vi "ReceiveFloat.vi"(6 "Timeout ms":i32=1, 7 "UDP Input":T1) -> (0 "Error Out":errorcluster, 1 "Received Data":dbl, 2 "Did Receive":bool, 3 "UDP Output":T1)   [LabVIEW 2019]
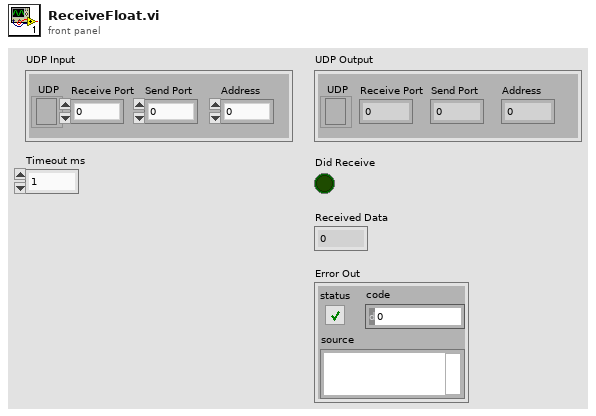
[diagram p1: front panel]
types:
  T1 = cluster{"UDP":refnum<k16>, "Receive Port":i32, "Send Port":i32, "Address":i64}
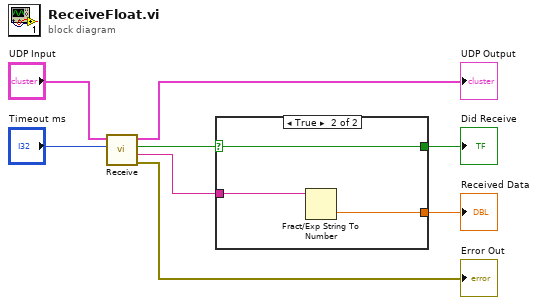
[diagram p0: block diagram]
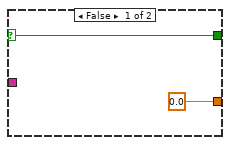
[diagram p2: hidden frame]
diagram:
  n1 = call "Receive.vi"("Timeout ms"="Timeout ms", "UDP Input"="UDP Input") -> ("Error Out"=→"Error Out":errorcluster, "Received Data"=w5:string, "Did Receive"=w2:bool, "UDP Output"=→"UDP Output":T1)  [unwired: 2 in]
  n2 = case shown="True" w2 {
    selector: w2 -> [w10 w11]
    tunnel: w5 -> [_ w13]
    tunnel: [0.0 w12] -> w4
    tunnel: [w10 w11] -> w1
    frame False {
    }
    frame True {
      n3 = Fract/Exp String To Number(string=w13) -> (number=w12:dbl)  [unwired: 3 in, 1 out]
    }
  }
  "Received Data" <- w4
  "Did Receive" <- w1
